vi "Messungaufnehmen_test.vi"() -> ()   [LabVIEW 2016]
uses:
  <vilib>/Waveform/WDTOps.llb/WDT Append Waveforms DBL.vi
  <vilib>/Waveform/WDTOps.llb/WDT Waveform Duration DBL.vi
  <vilib>/Waveform/WDTFileIO.llb/Export Waveform To Spreadsheet File.vi
panel:
  out "Waveform Data 2":waveform(dbl)(graph)
  out "Error_out":errorcluster
  in  "stop":bool
  out "t0":timestamp
  out "dt":dbl
  out "Y":dbl[](array[numeric])
  in  "VISA Name OZ in(OZ)":refnum<visa-resource-name>="USB0::0x0957::0x179B::MY54313507::INSTR"
  out "HardwareAntwort":string
  in  "Timeout (10000)":u32=10000
  out "error out":errorcluster
  out "VISA resource name out":refnum<visa-resource-name>
  in  "error in (no error)":errorcluster
  in  "Source Channel (0: Channel 1)":i32(ring) items=["Channel 1"=0, "Channel 2"=1, "Channel 3"=2, "Channel 4"=3, "Waveform Memory 1"=5, "Waveform Memory 2"=6, "Serial Bus 1"=7, "Serial Bus 2"=8, "Digital Bus Low"=9, "Digital Bus High "=10, "Digital Bus 1"=11, "Digital Bus 2"=12, "Function 1"=32, "Function 2"=33, "Function 3"=34, "Function 4"=35, "Math 1"=36, "Math 2"=37, "Math 3"=38, "Math 4"=39]
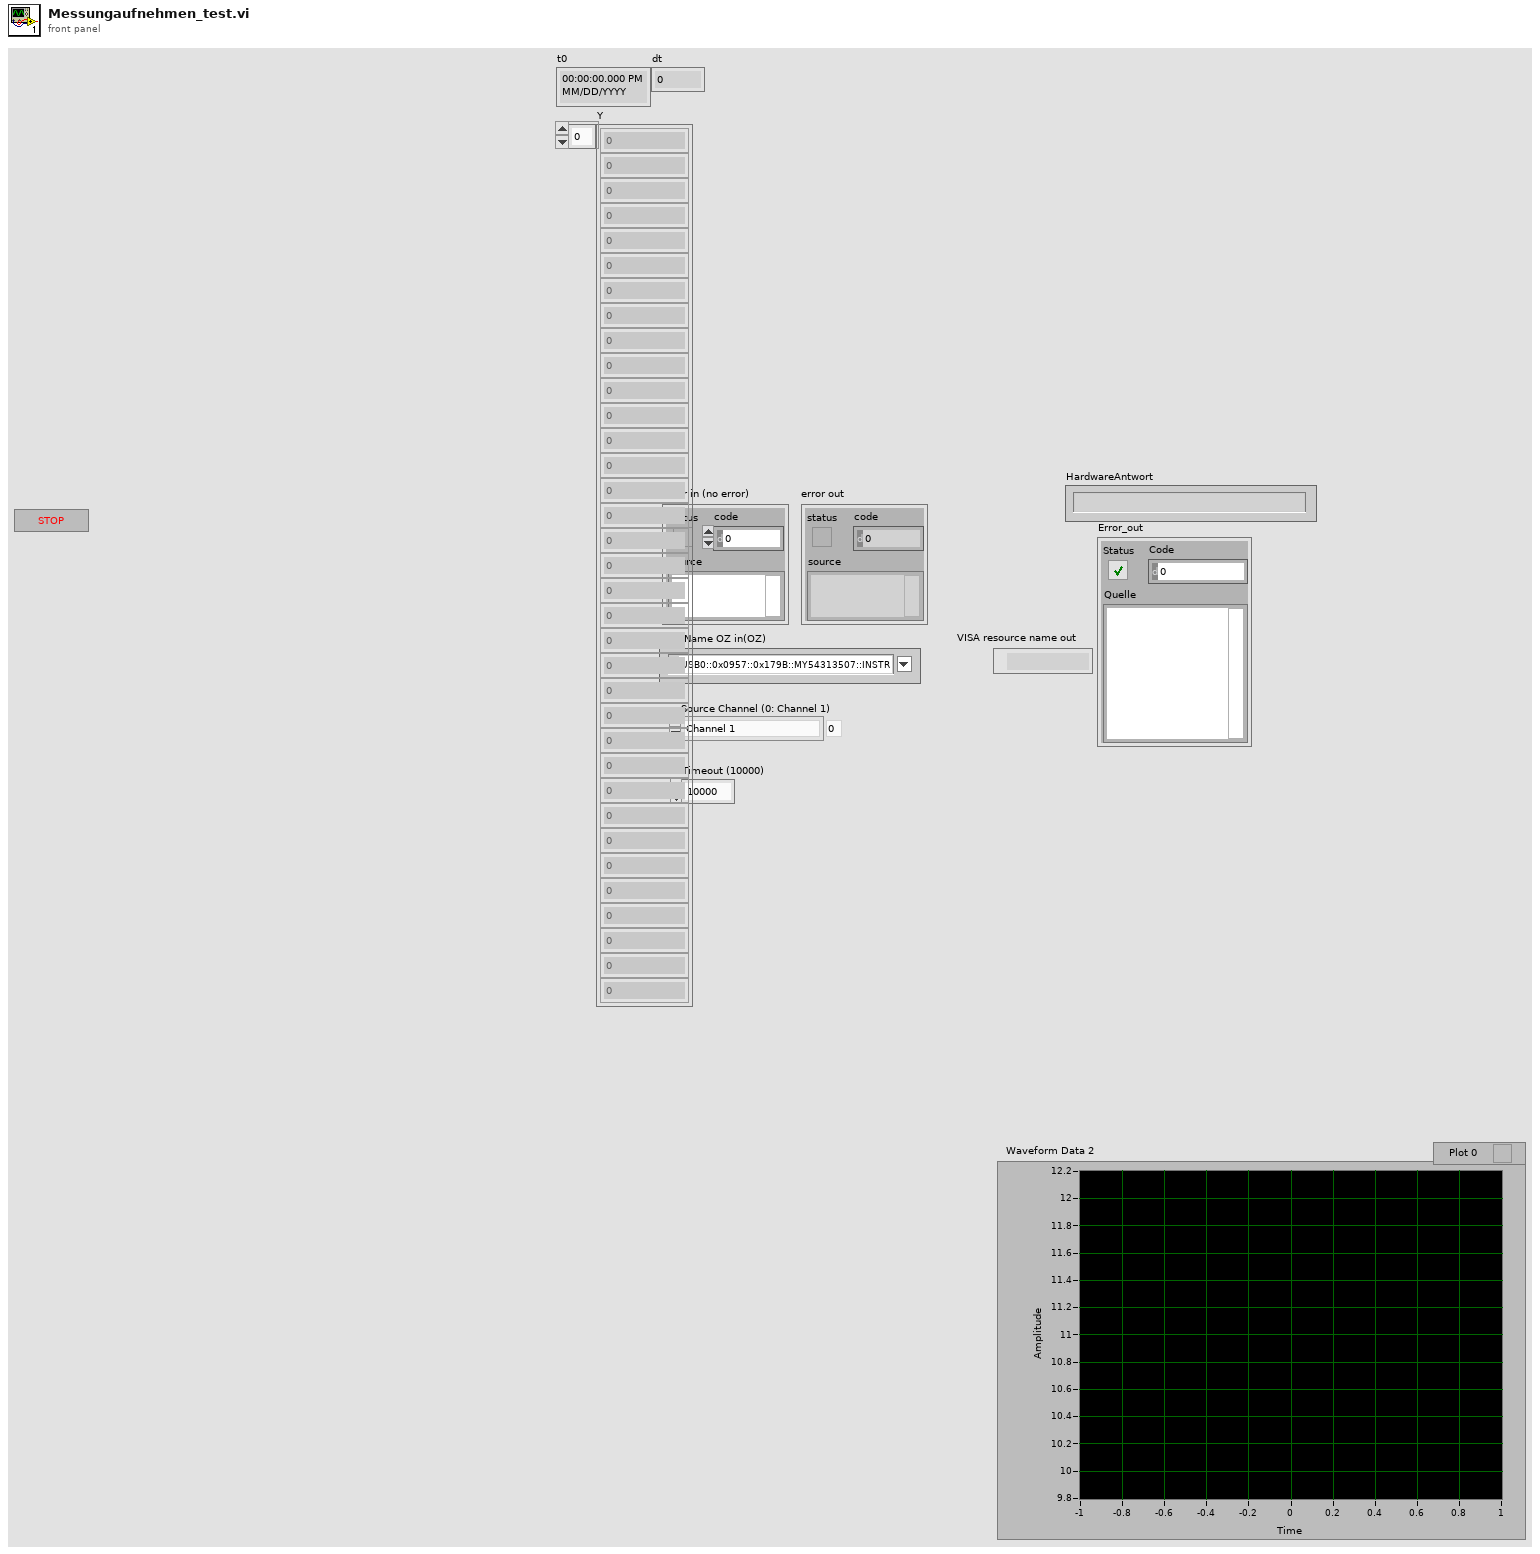
[diagram p1: front panel]
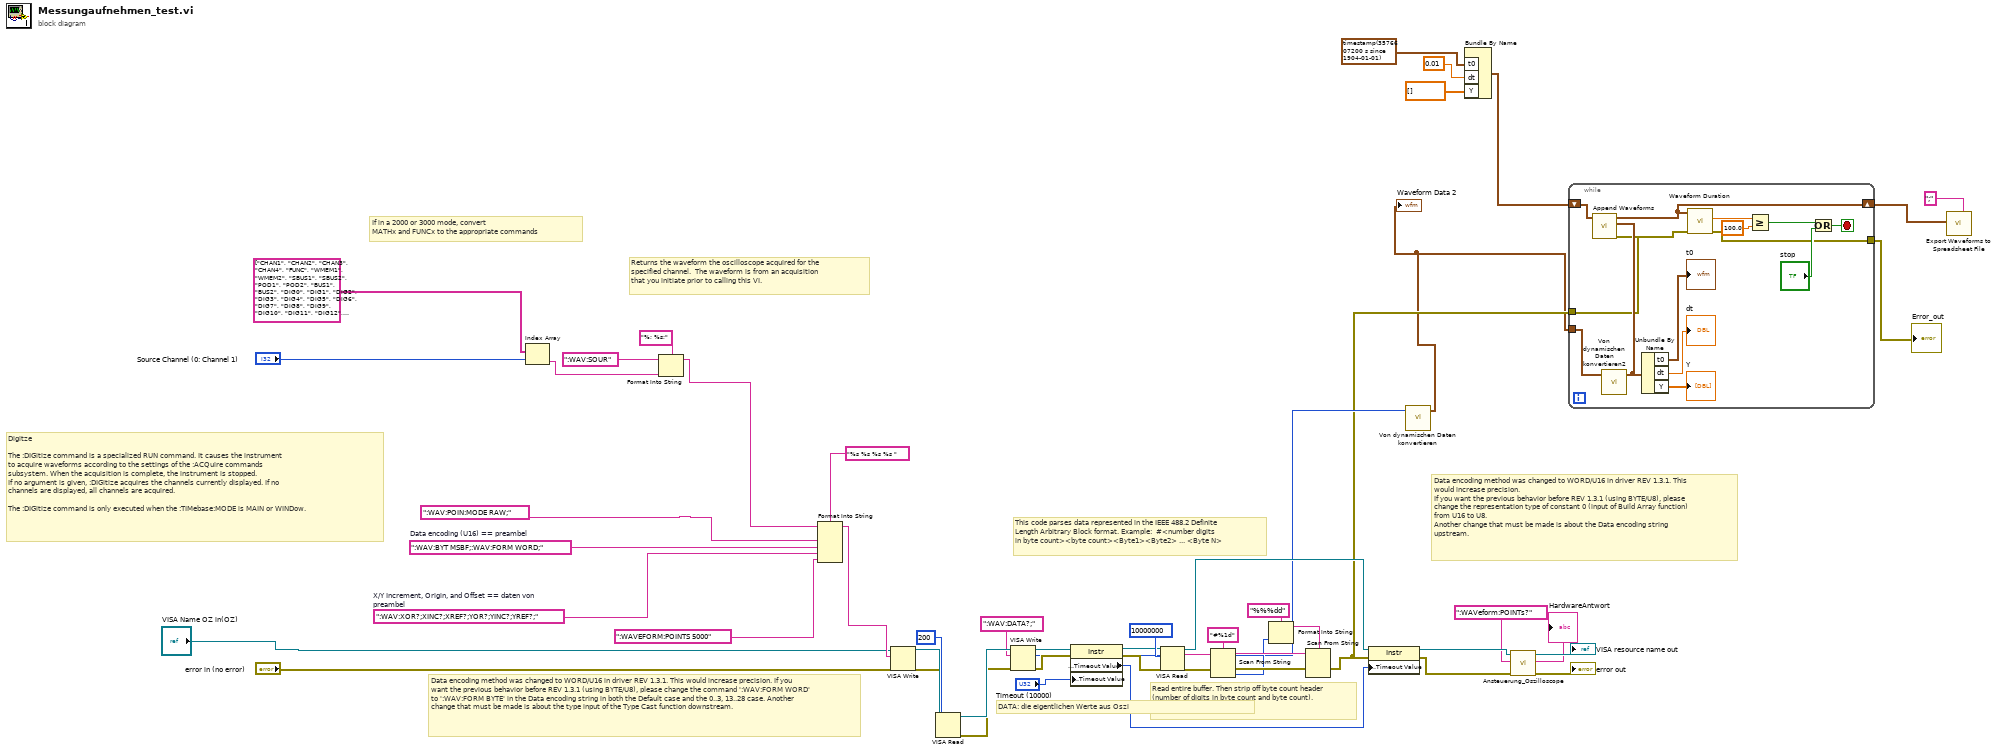
[diagram p0: block diagram]
diagram:
  w14 = ":WAV:XOR?;XINC?;XREF?;YOR?;YINC?;YREF?;"  # X/Y Increment, Origin, and Offset == daten von preambel
  w27 = ":WAV:BYT MSBF;:WAV:FORM WORD;"  # Data encoding (U16) == preambel
  # "DATA: die eigentlichen Werte aus Oszi"
  # "Digitze\n\nThe :DIGitize command is a specialized RUN command. It causes the instrument\nto acquire waveforms according to the settings of the :ACQuire commands\nsubsystem. When the acquisition is complete, the instrument is stopped.\nIf no argument is given, :DIGitize acquires the channels currently displayed. If no\nchannels are displayed, all channels are acquired.\n\nThe :DIGitize command is only executed when the :TIMebase:MODE is MAIN or WINDow."
  # "Data encoding method was changed to WORD/U16 in driver REV 1.3.1. This would increase precision. If you want the previous behavior before REV 1.3.1 (using BYTE/U8), please change the command ':WAV:FORM WORD' to ':WAV:FORM BYTE' in the Data encoding string in both the Default case and the 0..3, 13..28 case. Another change that must be made is about the type input of the Type Cast function downstream."
  # "Data encoding method was changed to WORD/U16 in driver REV 1.3.1. This would increase precision. \nIf you want the previous behavior before REV 1.3.1 (using BYTE/U8), please change the representation type of constant 0 (input of Build Array function) from U16 to U8. \nAnother change that must be made is about the Data encoding string upstream."
  # "If in a 2000 or 3000 mode, convert\nMATHx and FUNCx to the appropriate commands"
  # "Read entire buffer. Then strip off byte count header (number of digits in byte count and byte count)."
  # "This code parses data represented in the IEEE 488.2 Definite \nLength Arbitrary Block format. Example:  #<number digits \nin byte count><byte count><Byte1><Byte2> ... <Byte N>"
  # "Returns the waveform the oscilloscope acquired for the \nspecified channel.  The waveform is from an acquisition \nthat you initiate prior to calling this VI."
  n1 = Index Array(array=string[] ["CHAN1", "CHAN2", "CHAN3", "CHAN4", "FUNC", "WMEM1", "WMEM2", "SBUS1", "SBUS2", "POD1", "POD2", "BUS1", "BUS2", "DIG0", "DIG1", "DIG2", "DIG3", "DIG4", "DIG5", "DIG6", "DIG7", "DIG8", "DIG9", "DIG10", "DIG11", "DIG12", "DIG13", "DIG14", "DIG15", "EXT", "LINE", "WGEN", "FUNC1", "FUNC2", "FUNC3", "FUNC4", "MATH1", "MATH2", "MATH3", "MATH4"], index="Source Channel (0: Channel 1)") -> (element=w22:string)
  n2 = Format Into String(format string="%; %s;", initial string=":WAV:SOUR" ("Eingangs-String"), w22) -> (resulting string=w25:string)  [unwired: 1 in, 1 out]
  n3 = Format Into String(format string="%s %s %s %s ", initial string=w25, ":WAV:POIN:MODE RAW;", w27, w14, ":WAVEFORM:POINTS 5000" ("Eingang 4")) -> (resulting string=w26:string)  [unwired: 1 in, 1 out]
  n4 = VISA Write(VISA resource name="VISA Name OZ in(OZ)", write buffer=w26, error in (no error)="error in (no error)") -> (VISA resource name out=w32:refnum<visa-resource-name>, error out=w31:errorcluster)  [unwired: 1 out]
  n5 = VISA Read(VISA resource name=w32, byte count=u32 200, error in (no error)=w31) -> (VISA resource name out=w40:refnum<visa-resource-name>, error out=w39:errorcluster)  [unwired: 2 out]
  n6 = VISA Write(VISA resource name=w40, write buffer=":WAV:DATA?;", error in (no error)=w39) -> (VISA resource name out=w41:refnum<visa-resource-name>, return count=w10:u32, error out=w42:errorcluster)
  n7 = property class="Instr"(reference=w41, error in=w42, "General Settings:Timeout Value"="Timeout (10000)") -> (reference out=w36:refnum<visa-resource-name>, error out=w35:errorcluster, "General Settings:Timeout Value"=w38:u32)
  n8 = VISA Read(VISA resource name=w36, byte count=u32 10000000, error in (no error)=w35) -> (VISA resource name out=w34:refnum<visa-resource-name>, read buffer=w45:string, error out=w43:errorcluster)  [unwired: 1 out]
  n9 = Scan From String(format string="#%1d", input string=w45, error in=w43) -> (remaining string=w49:string, error out=w47:errorcluster, output 1=w46:i32)  [unwired: 1 in, 2 out]
  n10 = Format Into String(format string="%%%dd", w46) -> (resulting string=w48:string)  [unwired: 2 in, 1 out]
  n11 = Scan From String(format string=w48, input string=w49, error in=w47) -> (error out=w3:errorcluster)  [unwired: 1 in, 4 out]
  n12 = property class="Instr"(reference=w34, error in=w3, "General Settings:Timeout Value"=w38) -> (reference out=w19:refnum<visa-resource-name>, error out=w11:errorcluster)
  n13 = call "Von dynamischen Daten konvertieren"("Dynamic Data Type"=w10) -> ("Waveform"=w1:waveform(dbl))  [unwired: 3 in]
  "Waveform Data 2" <- w1
  n14 = Bundle By Name("t0"=timestamp(3576607200 s since 1904-01-01), "dt"=0.01, "Y"=dbl[] []) -> (w6:waveform(dbl))  [unwired: 1 in]
  n15 = call "Ansteuerung_Oszilloscope.vi"("Error_in"=w11, "Eingangs-String"=":WAVeform:POINTs?" ("format string"), "VISA Name OZ in(OZ)"=w19) -> ("Error_out"=→"error out":errorcluster, "Ausgangs-String"=→"HardwareAntwort":string, "VISA Name OZ out"=→"VISA resource name out":refnum<visa-resource-name>)  [unwired: 6 in]
  n16 = while {
    shift-right: [w62] -> w2
    shift-left: w6 -> [w64]
    tunnel: w1 -> [w53]
    tunnel: w3 -> [w54]
    tunnel: [w55] -> w4
    stop <- w57 stop-if-true
    n17 = call "Von dynamischen Daten konvertieren2"("Dynamic Data Type"=w53) -> ("Waveform"=w63:waveform(dbl))  [unwired: 3 in]
    n18 = call-poly <vilib>:"Append Waveforms.vi"("error in (no error)"=w54, "waveform B"=w63, "waveform A"=w64) -> ("error out"=w56:errorcluster, "waveform out"=w62:waveform(dbl))  [unwired: 7 in]
    n19 = Unbundle By Name(w63) -> ("t0"=→"t0":timestamp, "dt"=→"dt":dbl, "Y"=→"Y":dbl[])
    n20 = call-poly <vilib>:"Waveform Duration.vi"("error in (no error)"=w56, "waveform in"=w62) -> ("error out"=w55:errorcluster, "duration"=w61:dbl)  [unwired: 7 in, 1 out]
    n21 = Greater Or Equal?(x=w61, y=100.0) -> (x >= y?=w58:bool)
    n22 = Or(x=w58, y="stop") -> (x .or. y?=w57:bool)
  }
  "Error_out" <- w4
  n23 = call-poly <vilib>:"Export Waveforms to Spreadsheet File.vi"("delimiter (Tab)"=";", "waveform"=w2) -> ()  [unwired: 8 in, 2 out]
